vi "CoPilot Analyze.vi"(11 "JoystickDevRef":T1) -> (0 "La Fire at will?":bool, 1 "Ejection":bool, 2 "Suction":bool, 3 "Aim?":bool, 4 "Feeder?":bool, 5 "Elevation":dbl, 7 "Shoot Motors":dbl)   [LabVIEW 2012]
uses:
  <vilib>/Rock Robotics/WPI/Joystick/WPI_JoystickDevRef.ctl
  <vilib>/Rock Robotics/WPI/Joystick/WPI_JoystickDeviceEnum.ctl
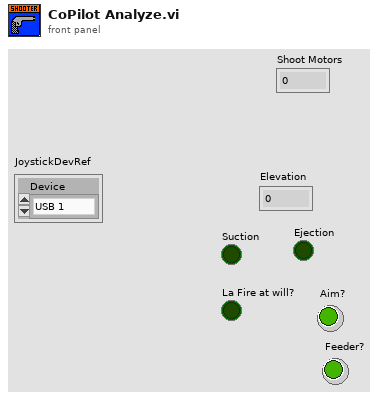
[diagram p1: front panel]
types:
  T1 = typedef "WPI_JoystickDevRef.ctl" = cluster{"Device":T2}
  T2 = typedef "WPI_JoystickDeviceEnum.ctl" = enum16{"USB 1", "USB 2", "USB 3", "USB 4", "Kinect 1", "Kinect 2"}
  T3 = typedef "WPI_JoystickButtonState.ctl" = cluster{"Button 1":bool, "Button 2":bool, "Button 3":bool, "Button 4":bool, "Button 5":bool, "Button 6":bool, "Button 7":bool, "Button 8":bool, "Button 9":bool, "Button 10":bool, "Button 11":bool, "Button 12":bool}
  T4 = cluster{"axis 1 (x)":dbl, "axis 2 (y)":dbl, "axis 3 (throttle)":dbl, "axis 4":dbl, "axis 5":dbl, "axis 6":dbl}
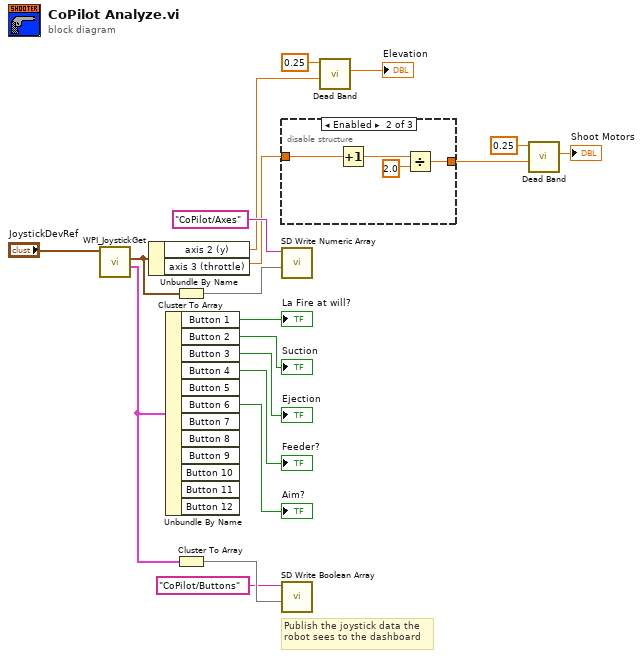
[diagram p0: block diagram]
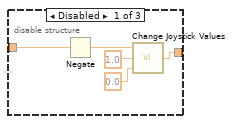
[diagram p2: hidden frame]
diagram:
  # "Publish the joystick data the\nrobot sees to the dashboard"
  n1 = call <vilib>:"WPI_JoystickGet.vi"("JoystickDevRef"="JoystickDevRef") -> ("Buttons"=w13:T3, "Axes"=w14:T4)  [unwired: 4 in, 1 out]
  n2 = Unbundle By Name(w14) -> ("axis 2 (y)"=w8:dbl, "axis 3 (throttle)"=w4:dbl)
  n3 = Unbundle By Name(w13) -> ("Button 1"=→"La Fire at will?":bool, "Button 2"=→"Suction":bool, "Button 3"=→"Ejection":bool, "Button 4"=→"Feeder?":bool, "Button 6"=→"Aim?":bool)  [unwired: 7 out]
  n4 = Cluster To Array(cluster=w14) -> (array=w16:dbl[])
  n5 = Cluster To Array(cluster=w13) -> (array=w18:bool[])
  n6 = disable-structure shown="Enabled" {
    disable-tunnel: w4 -> [w21 w28 w29]
    disable-tunnel: [w24 w25 w29] -> w3
    frame Disabled {
      n7 = Negate(x=w21) -> (-x=w20:dbl)
      n8 = call "Change Joystick Values.vi"("Change -1 to?"=0.0, "Change 1 to?"=1.0, "Joystick Input"=w20) -> ("Output Value"=w24:dbl)
    }
    frame Enabled {
      n9 = Increment(x=w28) -> (x+1=w27:dbl)
      n10 = Divide(x=w27, y=2.0) -> (x/y=w25:dbl)
    }
    frame Disabled {
    }
  }
  n11 = call <vilib>:"SD Write Numeric Array.vi"("Numeric Array"=w16, "Name"="CoPilot/Axes") -> ()  [unwired: 8 in, 2 out]
  n12 = call <vilib>:"SD Write Boolean Array.vi"("Boolean Array"=w18, "Name"="CoPilot/Buttons") -> ()  [unwired: 8 in, 2 out]
  n13 = call "Dead Band.vi"("Axis In"=w8, "Dead Band"=0.25) -> ("Axis Out"=→"Elevation":dbl)  [unwired: 9 in]
  n14 = call "Dead Band.vi"("Axis In"=w3, "Dead Band"=0.25) -> ("Axis Out"=→"Shoot Motors":dbl)  [unwired: 9 in]
